vi "차이 보고용.vi"() -> ()   [LabVIEW 2020]
panel:
  out "입력 값":dbl
  out "XY Graph":cluster{"Y":dbl[], "Y":dbl[]}[](graph) caption="입력값이 0~ 2까지 변동시 각 장비의 출력값의 변화"
  out "DTS-C 결과":dbl
  out "KDN-DTS 결과":dbl
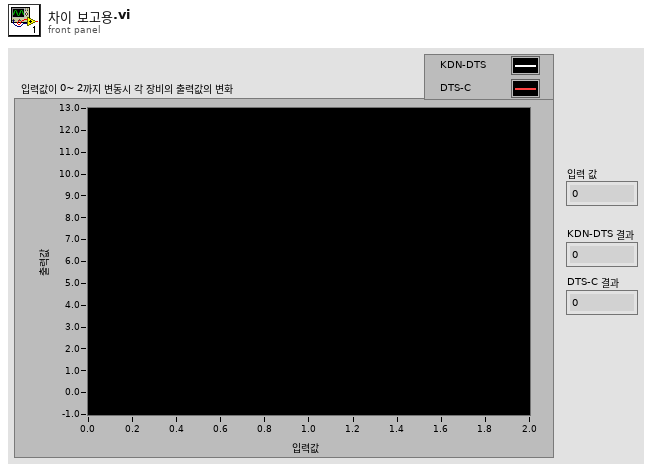
[diagram p1: front panel]
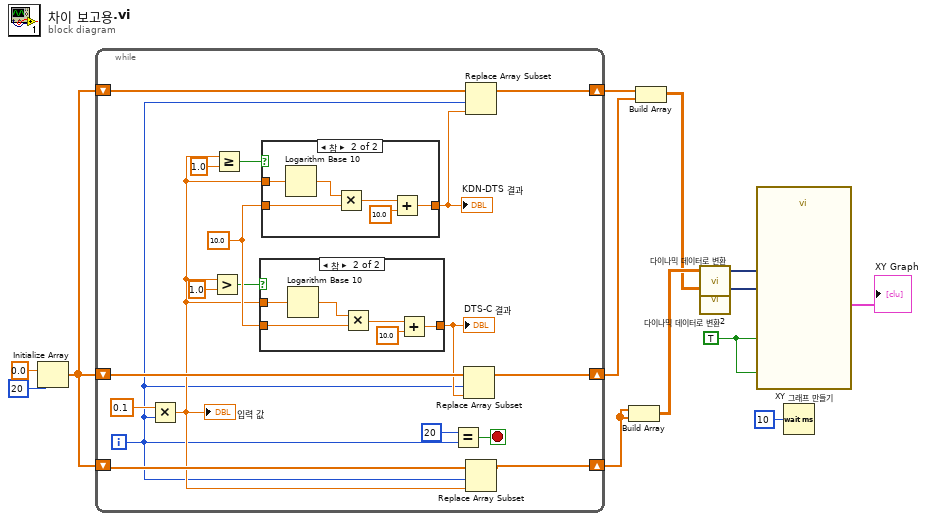
[diagram p0: block diagram]
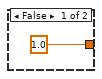
[diagram p2: hidden frame]
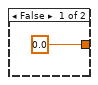
[diagram p3: hidden frame]
diagram:
  w3 = TRUE ("Reset")
  n1 = Initialize Array(0.0 ("원소"), 20 ("차원 크기")) -> (w10:dbl[])
  n2 = while {
    shift-right: [w19] -> w11
    shift-left: w10 -> [w20]
    shift-right: [w22] -> w12
    shift-left: w10 -> [w23]
    shift-right: [w17] -> w9
    shift-left: w10 -> [w16]
    i -> [w14]
    stop <- w24 stop-if-true
    w31 = 10.0 ("y")
    n3 = Multiply(x=0.1, y=w14) -> (x*y=w15:dbl)
    "입력 값" <- w15
    n4 = Greater?(x=w15, y=1.0) -> (0:w28:bool)
    n5 = Greater Or Equal?(x=w15, y=1.0) -> (x >= y?=w30:bool)
    n6 = case shown="참" w28 {
      tunnel: w15 -> [_ w38]
      tunnel: w31 -> [_ w36]
      tunnel: [1.0 w34] -> w18
      frame False {
      }
      frame True {
        n7 = Logarithm Base 10(1:w38) -> (0:w37:dbl)
        n8 = Multiply(x=w37, y=w36) -> (x*y=w33:dbl)
        n9 = Add(x=w33, y=10.0) -> (x+y=w34:dbl)
      }
    }
    "DTS-C 결과" <- w18
    n10 = case shown="참" w30 {
      tunnel: w15 -> [_ w45]
      tunnel: w31 -> [_ w43]
      tunnel: [0.0 w42] -> w21
      frame False {
      }
      frame True {
        n11 = Logarithm Base 10(1:w45) -> (0:w44:dbl)
        n12 = Multiply(x=w44, y=w43) -> (x*y=w41:dbl)
        n13 = Add(x=w41, y=10.0) -> (x+y=w42:dbl)
      }
    }
    "KDN-DTS 결과" <- w21
    n14 = Equal?(x=20, y=w14) -> (x = y?=w24:bool)
    n15 = Replace Array Subset(array=w20, new element=w18, index=w14) -> (w19:dbl[])
    n16 = Replace Array Subset(array=w23, new element=w21, index=w14) -> (w22:dbl[])
    n17 = Replace Array Subset(array=w16, new element=w15, index=w14) -> (w17:dbl[])
  }
  n18 = Build Array(w9, w9) -> (w7:dbl[][])
  n19 = Build Array(w12, w11) -> (w5:dbl[][])
  n20 = call "다이나믹 데이터로 변환"("2D Array"=w7) -> ("Dynamic Data Type"=w6:dynamicdata)  [unwired: 3 in]
  n21 = call "다이나믹 데이터로 변환2"("2D Array"=w5) -> ("Dynamic Data Type"=w4:dynamicdata)  [unwired: 3 in]
  n22 = call "XY 그래프 만들기"("Enable"=w3, "Reset"=w3, "Y Input"=w4, "X Input"=w6) -> ("XY Graph"=→"XY Graph":cluster{"X":dbl[], "Y":dbl[]}[])  [unwired: 6 in, 1 out]
  n23 = Wait (ms)(milliseconds to wait=u32 10 ("대기 시간 (ms)")) -> ()  [unwired: 1 out]
